vi "Update Meas Type to J-t Scan.vi"(11 "Cell details array in":T1(array[cluster])) -> (3 "Cell details array out":T1(array[cluster]))   [LabVIEW 2016]
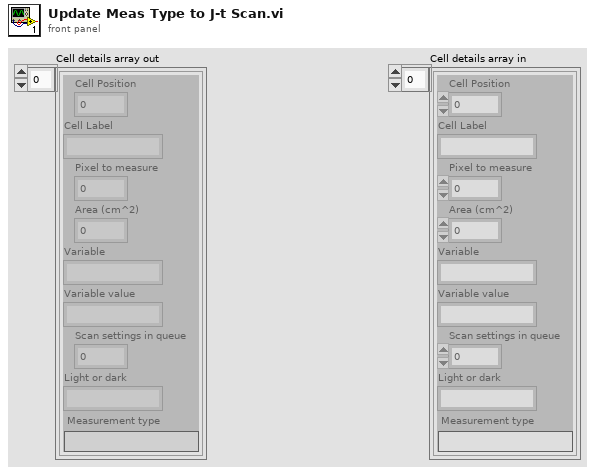
[diagram p1: front panel]
types:
  T1 = cluster{"Cell Position":i32, "Cell Label":string, "Pixel to measure":u16, "Area (cm^2)":dbl, "Variable":string, "Variable value":string, "Scan settings in queue":u16, "Light or dark":string, "Measurement type":string}[]
  T2 = cluster{"Cell Position":i32, "Cell Label":string, "Pixel to measure":u16, "Area (cm^2)":dbl, "Variable":string, "Variable value":string, "Scan settings in queue":u16, "Light or dark":string, "Measurement type":string}
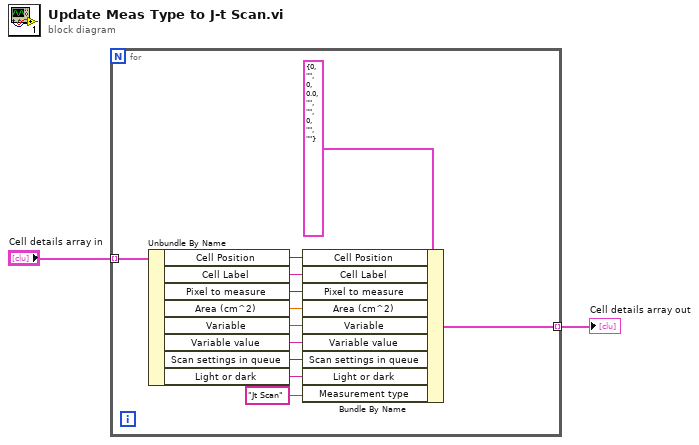
[diagram p0: block diagram]
diagram:
  n1 = for {
    tunnel: "Cell details array in" -> [w14] mode=indexing
    tunnel: [w3] -> w1 mode=indexing
    n2 = Unbundle By Name(w14) -> ("Cell Position"=w12:i32, "Cell Label"=w11:string, "Pixel to measure"=w10:u16, "Area (cm^2)"=w9:dbl, "Variable"=w8:string, "Variable value"=w7:string, "Scan settings in queue"=w6:u16, "Light or dark"=w5:string)
    n3 = Bundle By Name(cluster=T2 {"Cell Position"=0, "Cell Label"="", "Pixel to measure"=0, "Area (cm^2)"=0.0, "Variable"="", "Variable value"="", "Scan settings in queue"=0, "Light or dark"="", "Measurement type"=""} ("Cluster"), "Cell Position"=w12, "Cell Label"=w11, "Pixel to measure"=w10, "Area (cm^2)"=w9, "Variable"=w8, "Variable value"=w7, "Scan settings in queue"=w6, "Light or dark"=w5, "Measurement type"="Jt Scan") -> (w3:T2)
  }
  "Cell details array out" <- w1
